vi "ABCSecondKicker.vi"(6 "Tactic index in":i32, 7 "first call":bool, 8 "error in (no error) 2":errorcluster, 10 "Game in":refnum<class "Game.lvclass">, 11 "ABCSecondKicker in":refnum<class "ABCSecondKicker.lvclass">) -> (0 "error out 2":errorcluster, 1 "Robot out":refnum<class "Robot.lvclass">, 2 "tactic index":i32, 3 "ABCSecondKicker out":refnum<class "ABCSecondKicker.lvclass">)   [LabVIEW 2023, in "ABCSecondKicker.lvclass"]
uses:
  ABCSecondKicker.lvclass
  C:/Users/ebert/Desktop/roboime/SSL_AI/Role_class/Role.lvclass
  Game_class/Game.lvclass
  Robot_class/Robot.lvclass
  Role_class/Role.lvclass/Role.ctl
  Tacticbook_class/Tacticbook.lvclass/Tacticbook.ctl
  KickToPassReceiverTactic_class/KickToPassReceiverTacticStates.ctl
  KickToPassReceiverTactic_class/KickToPassReceiverTactic.lvclass/KickToPassReceiverTactic.ctl
  Tacticbook_class/Read WaitPassTactic.vi
  Tacticbook_class/Write WaitPassTactic.vi
  KickToPassReceiverTactic_class/Read States.vi
  Role_class/Read Tacticbook.vi
  Role_class/Write Tacticbook.vi
  Role_class/Write tactic_index.vi
  Role_class/Read RobotRef.vi
  Tacticbook_class/Tacticbook.lvclass
  WaitPassTactic_class/WaitPassTactic.lvclass
  KickToPassReceiverTactic_class/KickToPassReceiverTactic.lvclass
  PassObserverTactic_class/PassObserverTactic.lvclass
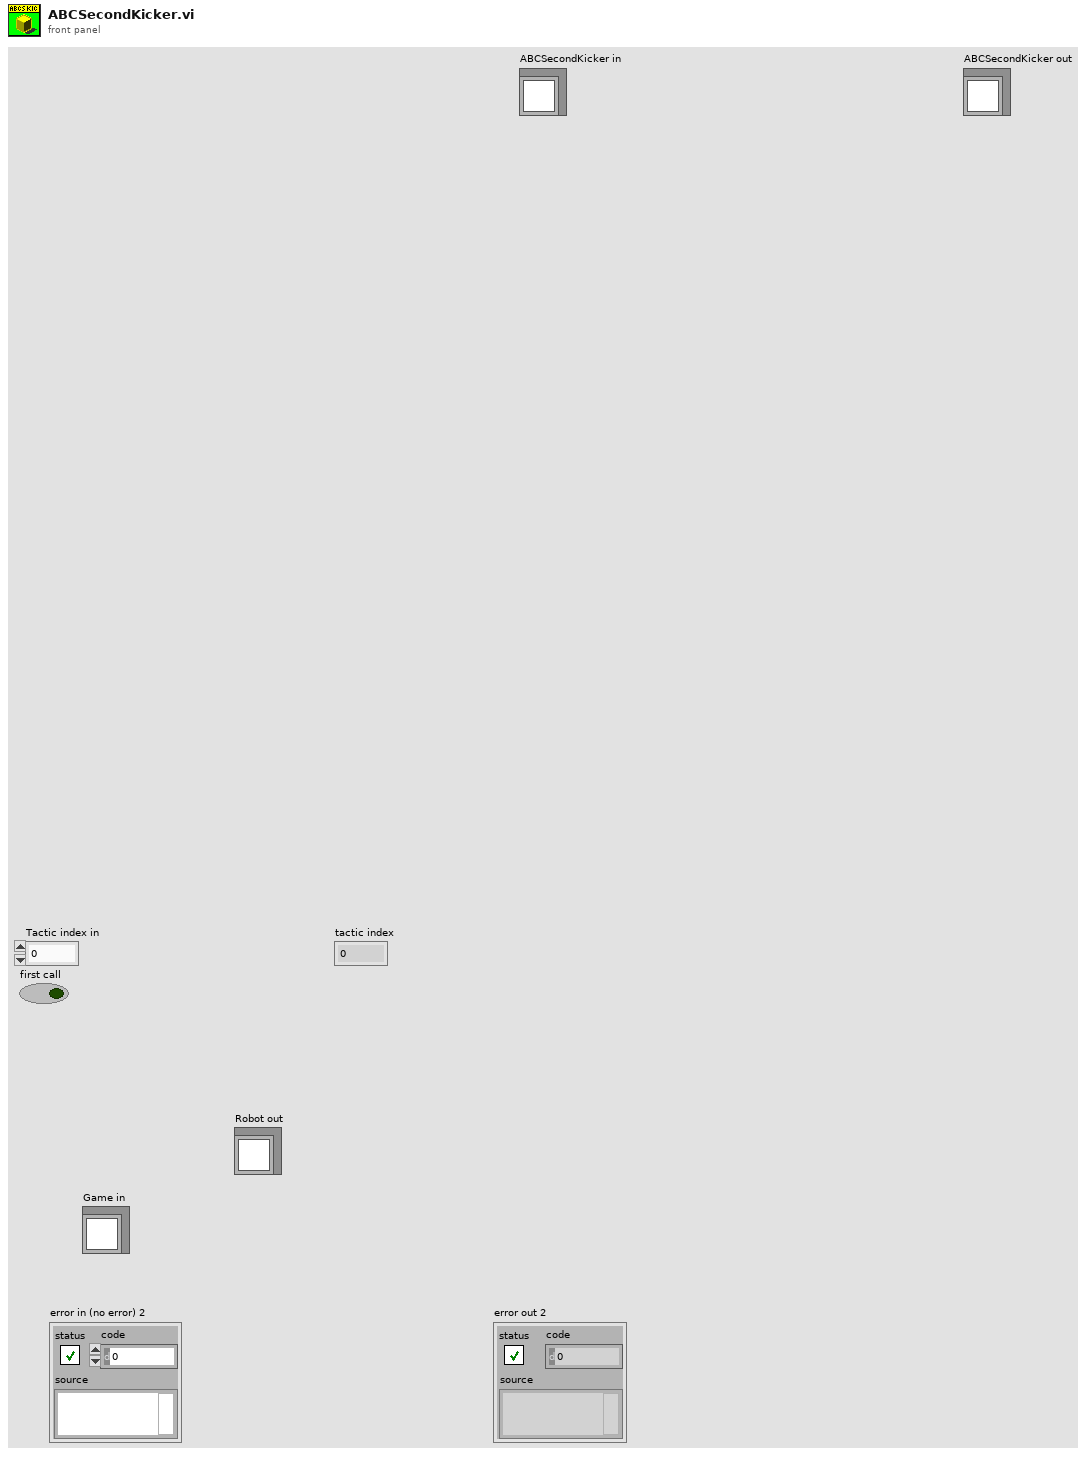
[diagram p1: front panel]
types:
  T1 = typedef "KickToPassReceiverTacticStates.ctl" = enum16{"Halt", "GoToReceiveTable", "KickToPassReceiver", "WaitPass", "Exit"}
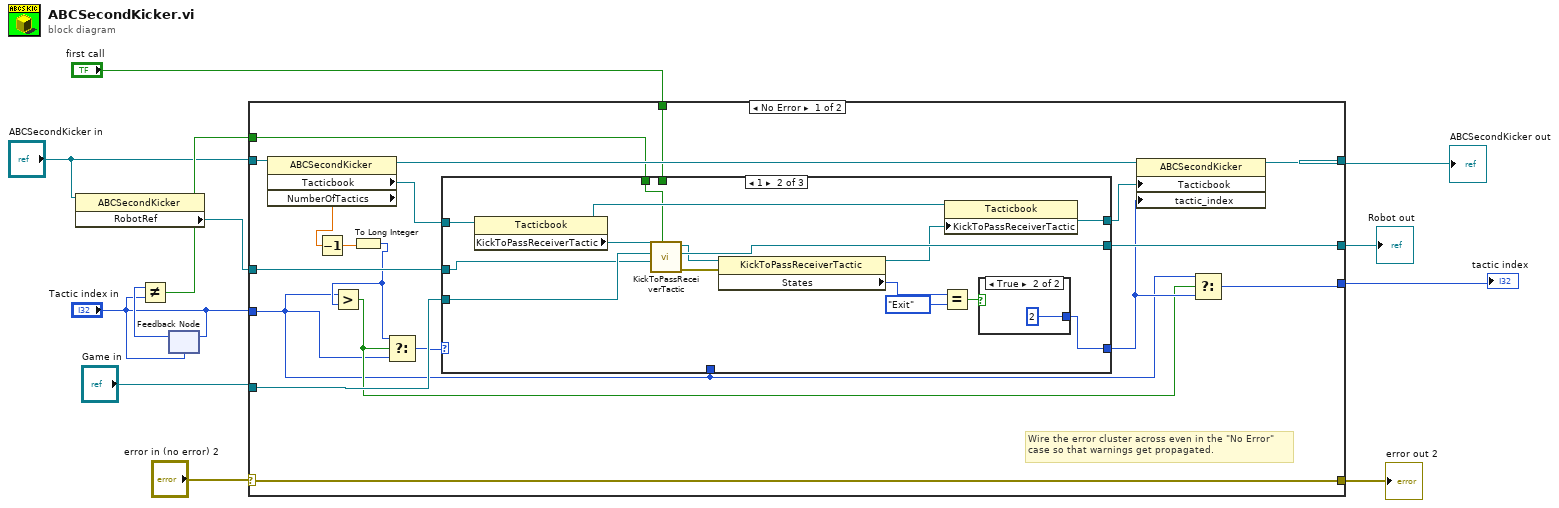
[diagram p0: block diagram]
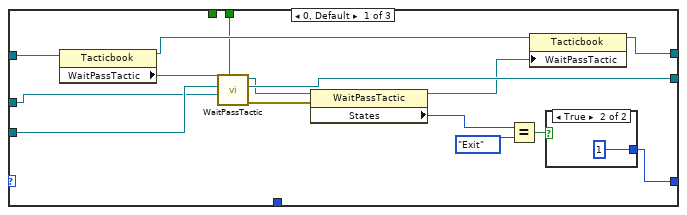
[diagram p2: hidden frame]
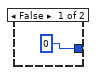
[diagram p3: hidden frame]
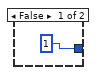
[diagram p4: hidden frame]
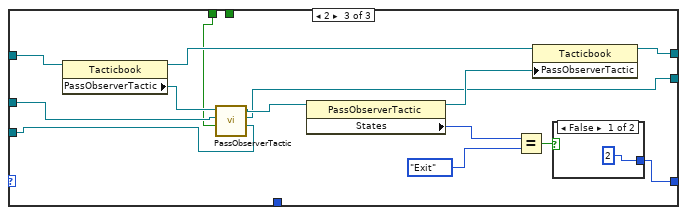
[diagram p5: hidden frame]
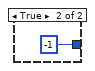
[diagram p6: hidden frame]
diagram:
  n1 = property class="ABCSecondKicker"(reference="ABCSecondKicker in") -> ("RobotRef"=w10:refnum<class "Robot.lvclass">)  [unwired: 1 in, 2 out]
  n2 = feedback #1("Tactic index in") -> (w6:i32)
  n3 = Not Equal?(x=w6, y="Tactic index in") -> (x != y?=w4:bool)
  n4 = feedback-in #1("Tactic index in") -> ()
  n5 = case shown="No Error" "error in (no error) 2" {
    selector: "error in (no error) 2" -> [w31 w84]
    tunnel: [w31 w84] -> w11
    tunnel: [w29 w83] -> w2
    tunnel: "ABCSecondKicker in" -> [w30 w83]
    tunnel: w10 -> [w26 w82]
    tunnel: [w25 w82] -> w3
    tunnel: "Game in" -> [w23 _]
    tunnel: [w21 _] -> w9
    tunnel: "Tactic index in" -> [w13 _]
    tunnel: "first call" -> [w17 _]
    tunnel: w4 -> [w14 _]
    frame No Error {
      # "Wire the error cluster across even in the \"No Error\"\ncase so that warnings get propagated."
      n6 = property class="ABCSecondKicker"(reference=w30) -> (reference out=w28:refnum<class "ABCSecondKicker.lvclass">, "Tacticbook"=w27:refnum<class "Tacticbook.lvclass">, "NumberOfTactics"=w18:dbl)  [unwired: 1 in, 1 out]
      n7 = Decrement(x=w18) -> (x-1=w16:dbl)
      n8 = To Long Integer(number=w16) -> (32bit integer=w15:i32)
      n9 = Greater?(x=w13, y=w15) -> (0:w19:bool)
      n10 = Select(t=w15, s=w19, f=w13) -> (s? t:f=w20:i32)
      n11 = case shown="1" w20 {
        tunnel: [w34 w51 w73] -> w22
        tunnel: w27 -> [w46 w63 w77]
        tunnel: w26 -> [w37 w54 w71]
        tunnel: [w45 w62 w68] -> w25
        tunnel: [w41 w58 w75] -> w24
        tunnel: w23 -> [w38 w55 w70]
        tunnel: w17 -> [w33 _ _]
        tunnel: w14 -> [_ w50 w66]
        tunnel: w13 -> [_ _ _]
        frame 0, Default {
          n12 = property class="Tacticbook"(reference=w46) -> (reference out=w43:refnum<class "Tacticbook.lvclass">, "WaitPassTactic"=w40:refnum<class "WaitPassTactic.lvclass">)  [unwired: 1 in, 1 out]
          n13 = call-dynamic "WaitPassTactic.vi"("first call"=w33, "Robot"=w37, "Game in"=w38, "WaitPassTactic in"=w40) -> ("error out"=w44:errorcluster, "Robot out"=w45:refnum<class "Robot.lvclass">, "WaitPassTactic out"=w39:refnum<class "WaitPassTactic.lvclass">)  [unwired: 5 in]
          n14 = property class="WaitPassTactic"(reference=w39, error in=w44) -> (reference out=w42:refnum<class "WaitPassTactic.lvclass">, "States"=w35:enum16{"State 0", "State 1", "State 2", "Exit"})  [unwired: 1 out]
          n15 = Equal?(x=w35, y=enum16{"State 0", "State 1", "State 2", "Exit"}."Exit") -> (x = y?=w36:bool)
          n16 = property class="Tacticbook"(reference=w43, "WaitPassTactic"=w42) -> (reference out=w41:refnum<class "Tacticbook.lvclass">)  [unwired: 1 in, 1 out]
          n17 = case shown="True" w36 {
            tunnel: [0 1] -> w34
            frame False {
            }
            frame True {
            }
          }
        }
        frame 1 {
          n18 = property class="Tacticbook"(reference=w63) -> (reference out=w60:refnum<class "Tacticbook.lvclass">, "KickToPassReceiverTactic"=w57:refnum<class "KickToPassReceiverTactic.lvclass">)  [unwired: 1 in, 1 out]
          n19 = call "KickToPassReceiverTactic.vi"("first call"=w50, "Robot"=w54, "Game in"=w55, "KickToPassReceiverTactic in"=w57) -> ("error out"=w61:errorcluster, "Robot out"=w62:refnum<class "Robot.lvclass">, "KickToPassReceiverTactic out"=w56:refnum<class "KickToPassReceiverTactic.lvclass">)  [unwired: 5 in]
          n20 = property class="KickToPassReceiverTactic"(reference=w56, error in=w61) -> (reference out=w59:refnum<class "KickToPassReceiverTactic.lvclass">, "States"=w52:T1)  [unwired: 1 out]
          n21 = Equal?(x=w52, y=KickToPassReceiverTacticStates."Exit") -> (x = y?=w53:bool)
          n22 = property class="Tacticbook"(reference=w60, "KickToPassReceiverTactic"=w59) -> (reference out=w58:refnum<class "Tacticbook.lvclass">)  [unwired: 1 in, 1 out]
          n23 = case shown="True" w53 {
            tunnel: [1 2] -> w51
            frame False {
            }
            frame True {
            }
          }
        }
        frame 2 {
          n24 = property class="Tacticbook"(reference=w77) -> (reference out=w76:refnum<class "Tacticbook.lvclass">, "PassObserverTactic"=w72:refnum<class "PassObserverTactic.lvclass">)  [unwired: 1 in, 1 out]
          n25 = call-dynamic "PassObserverTactic.vi"("Game in"=w70, "first call"=w66, "Robot"=w71, "PassObserverTactic in"=w72) -> ("Robot"=w68:refnum<class "Robot.lvclass">, "PassObserverTactic out"=w69:refnum<class "PassObserverTactic.lvclass">)  [unwired: 5 in, 1 out]
          n26 = property class="PassObserverTactic"(reference=w69) -> (reference out=w74:refnum<class "PassObserverTactic.lvclass">, "States"=w78:enum16{"PassObserver", "Halt", "Exit"})  [unwired: 1 in, 1 out]
          n27 = Equal?(x=w78, y=enum16{"PassObserver", "Halt", "Exit"}."Exit") -> (x = y?=w79:bool)
          n28 = property class="Tacticbook"(reference=w76, "PassObserverTactic"=w74) -> (reference out=w75:refnum<class "Tacticbook.lvclass">)  [unwired: 1 in, 1 out]
          n29 = case shown="False" w79 {
            tunnel: [2 -1] -> w73
            frame False {
            }
            frame True {
            }
          }
        }
      }
      n30 = property class="ABCSecondKicker"(reference=w28, "Tacticbook"=w24, "tactic_index"=w22) -> (reference out=w29:refnum<class "ABCSecondKicker.lvclass">)  [unwired: 1 in, 1 out]
      n31 = Select(t=w13, s=w19, f=w22) -> (s? t:f=w21:i32)
    }
    frame Error {
    }
  }
  "ABCSecondKicker out" <- w2
  "error out 2" <- w11
  "tactic index" <- w9
  "Robot out" <- w3
